vi "Settings.vi"() -> ()   [LabVIEW 2015]
panel:
  in  "Sensor Trigger Time (ms)":dbl
  in  "Speed Approaching and Crossing Drive Defense":dbl
  in  "Time Grabber Lowers Cheval":dbl
  in  "Speed Crossing Cheval":dbl
  in  "Speed Approaching Cheval":dbl
  in  "Min Turning Speed":dbl=2.0
  in  "Turn to Target Acceptable Error":dbl=2.0
  in  "Robot Jiggle Power":dbl=0.5
  in  "Robot Jiggle Frequency":i32=15
  in  "Robot Twist Deadband":dbl
  in  "Robot Twist Max Output":dbl
  in  "Robot Forward-Reverse Deadband":dbl
  in  "Robot Forward-Reverse Max Output":dbl
  in  "Left Grabber Lowered":dbl=779.0
  in  "Left Grabber Middle":dbl=1351.0
  in  "Left Grabber Raised":dbl=1830.0
  in  "Settings File Location":path=path "C:/ni-rt/startup/Settings.txt"
  in  "Motion Profile dt (ms)":dbl=40.0
  in  "Lower Safety Right":dbl=2902.0
  in  "Uncocked Upper Safety Right":dbl=1766.0
  in  "Upper Safety Right":dbl=2287.0
  in  "Lower Safety Left":dbl=779.0
  in  "Uncocked Upper Safety Left":dbl=1917.0
  in  "Upper Safety Left":dbl=227.0
  in  "Right Grabber Lowered":dbl=2902.0
  in  "Right Grabber Middle":dbl=2303.0
  in  "Right Grabber Raised":dbl=1803.0
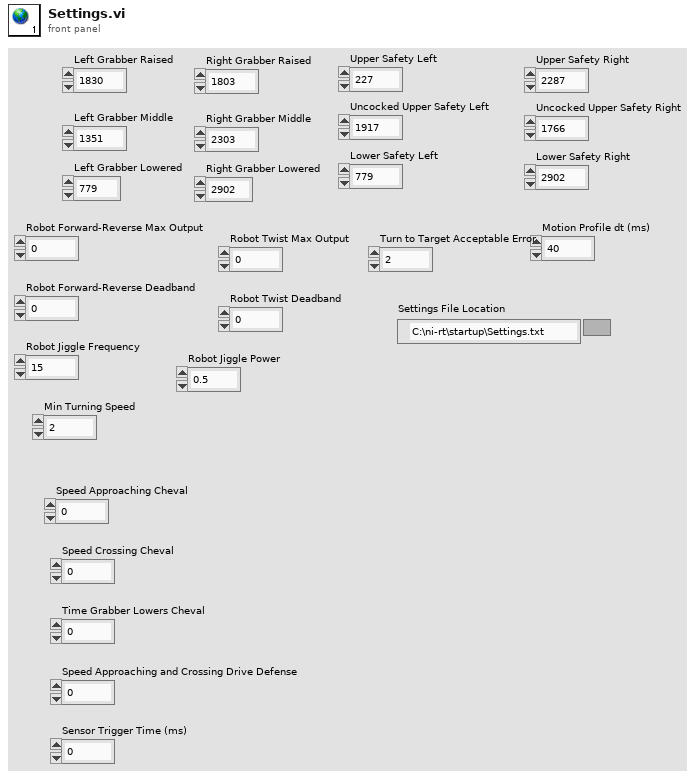
[diagram p1: front panel]
diagram:
